vi "SV Time-Varying Loudness_2014.vi"   [LabVIEW 2017, in "SoundVib_SoundQuality.lvlib"]
doc: "Computes time-varying loudness of the sound pressure signal from a time-varying 1/3 octave band spectrum."
uses:
  <vilib>/addons/Sound and Vibration/svt_Sound Quality/SoundVib_SoundQuality.lvlib
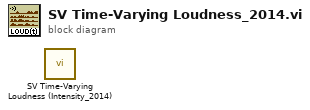
[diagram p0: block diagram]
diagram:
  n1 = call <vilib>:"SV Time-Varying Loudness (Intensity_2014).vi"() -> ()  [unwired: 11 in, 5 out]
